vi "GetElementIndices.vi"(6 "error in":errorcluster, 9 "NamedBundler in":refnum<class "NamedUnbundler.lvclass">) -> (0 "error out":errorcluster, 3 "NamedBundler out":refnum<class "NamedUnbundler.lvclass">, 4 "indices":string)   [LabVIEW 2014, in "Raspberry Pi Compatible Compiler for LabVIEW.lvlib" / "NamedUnbundler.lvclass"]
uses:
  NamedUnbundler.lvclass
  Python/Parsing/ListTypesTD.ctl
  Raspberry Pi Compatible Compiler for LabVIEW.lvlib
  Python/Parsing/Python Functions.lvlib
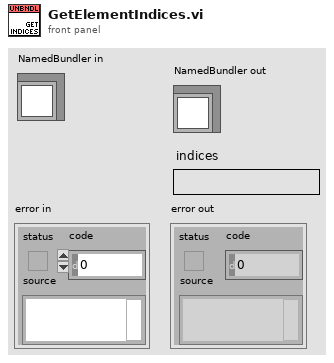
[diagram p1: front panel]
types:
  T1 = typedef "Raspberry Pi Compatible Compiler for LabVIEW.lvlib/Python Functions.lvlib/ListTypesTD.ctl" = enum16{"list", "tuple", "parameter list", "output list", "return values"}
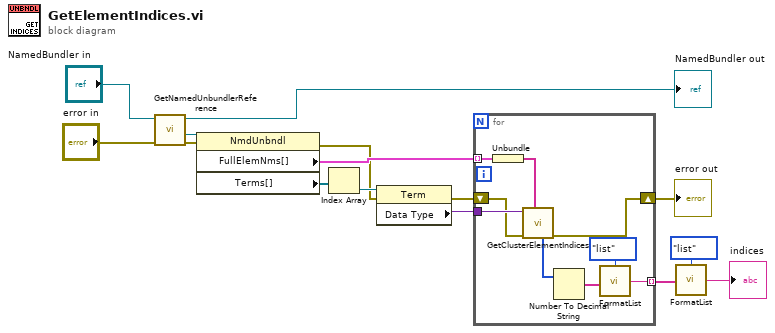
[diagram p0: block diagram]
diagram:
  n1 = call "GetNamedUnbundlerReference.vi"("error in"="error in", "NamedBundler in"="NamedBundler in") -> ("error out"=w12:errorcluster, "reference out"=w13:refnum<vi>, "NamedBundler out"=→"NamedBundler out":refnum<class "NamedUnbundler.lvclass">)  [unwired: 7 in]
  n2 = property class="NmdUnbndl"(reference=w13, error in=w12) -> (error out=w6:errorcluster, "FullElemNms[]"=w11:cluster{string[]}[], "Terms[]"=w10:refnum<vi>[])  [unwired: 1 out]
  n3 = Index Array(array=w10) -> (element=w9:refnum<vi>)  [unwired: 1 in]
  n4 = property class="Term"(reference=w9, error in=w6) -> (error out=w7:errorcluster, "Data Type"=w8:variant)  [unwired: 1 out]
  n5 = for {
    tunnel: w11 -> [w24] mode=indexing
    tunnel: w8 -> [w22]
    shift-right: [w20] -> w4
    shift-left: w7 -> [w21]
    tunnel: [w19] -> w3 mode=indexing
    n6 = Unbundle(w24) -> (w23:string[])
    n7 = call "GetClusterElementIndices.vi"("Element Name"=w23, "error in"=w21, "Cluster"=w22) -> ("error out"=w20:errorcluster, "indices"=w16:i32[])  [unwired: 5 in]
    n8 = Number To Decimal String(number=w16) -> (decimal integer string=w17:string[])  [unwired: 1 in]
    n9 = call "FormatList.vi"("values"=w17, "type"=ListTypesTD."list") -> ("python object"=w19:string)
  }
  "error out" <- w4
  n10 = call "FormatList.vi"("values"=w3, "type"=ListTypesTD."list") -> ("python object"=→"indices":string)
